vi "Restore Diagram Appearance.vi"(7 "Subpanel":refnum<vi>, 8 "error in (no error)":errorcluster, 9 "Bounds":T1, 10 "Origin":T2, 11 "Inserted VI":refnum<vi>) -> (0 "error out":errorcluster)   [LabVIEW 2020, in "Choose Implementation Dialog.lvlib"]
uses:
  Choose Implementation Dialog.lvlib
  <vilib>/Utility/miscctls.llb/LVPointTypeDef.ctl
  <vilib>/Utility/miscctls.llb/LVRectTypeDef.ctl
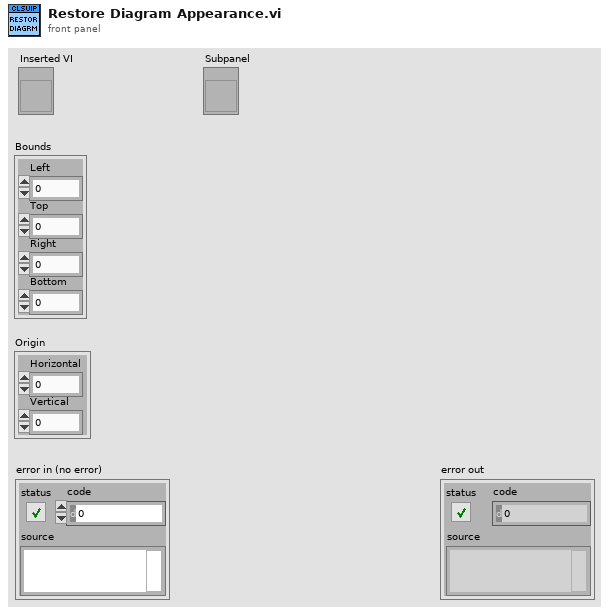
[diagram p1: front panel]
types:
  T1 = typedef "LVRectTypeDef.ctl" = cluster{"Left":i16, "Top":i16, "Right":i16, "Bottom":i16}
  T2 = typedef "LVPointTypeDef.ctl" = cluster{"Horizontal":i16, "Vertical":i16}
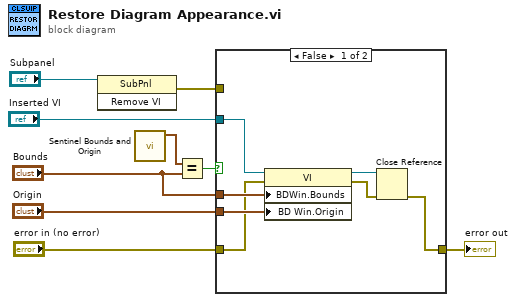
[diagram p0: block diagram]
diagram:
  n1 = invoke class="SubPnl" method="Remove VI"(reference="Subpanel") -> (error out=w2:errorcluster)  [unwired: 2 in, 2 out]
  n2 = call "Sentinel Bounds and Origin.vi"() -> ("Sentinel Bounds"=w1:T1)  [unwired: 10 in, 1 out]
  n3 = Equal?(x=w1, y="Bounds") -> (x = y?=w7:bool)
  n4 = case shown="False" w7 {
    tunnel: "Inserted VI" -> [w14 _]
    tunnel: "Bounds" -> [w15 _]
    tunnel: "Origin" -> [w16 _]
    tunnel: "error in (no error)" -> [w11 w17]
    tunnel: [w10 w17] -> w4
    tunnel: w2 -> [_ _]
    frame False {
      n5 = property class="VI"(reference=w14, error in=w11, "BDWin.Bounds"=w15, "BD Win.Origin"=w16) -> (reference out=w13:refnum<vi>, error out=w12:errorcluster)
      n6 = Close Reference(reference=w13, error in (no error)=w12) -> (error out=w10:errorcluster)
    }
    frame True {
    }
  }
  "error out" <- w4
